vi "MICSD Status.vi"(0 "VISA Resource Name":refnum<visa-resource-name>, 11 "error in (no error)":errorcluster) -> (3 "Data Status":T1={"TX_BlockCount"=2650, "RX_BlockCount"=2650, "DataErrorCount"=2650}, 4 "dup VISA Resource Name":refnum<visa-resource-name>, 6 "Status Flags":T4, 8 "Link Status":T3={"ImplantID"=0, "CompanyID"=0, "RF_Channel"=4, "RX_Mod"=0, "TX_Mod"=0, "TXBlockSize"=15, "RXBlockSize"=15, "BlocksPerPack"=31} {"BlocksPerPack" items=["1"=1, "2"=2, "3"=3, "4"=4, "5"=5, "6"=6, "7"=7, "8"=8, "9"=9, "10"=10, "11"=11, "12"=12, "13"=13, "14"=14, "15"=15, "16"=16, "17"=17, "18"=18, "19"=19, "20"=20, "21"=21, "22"=22, "23"=23, "24"=24, "25"=25, "26"=26, "27"=27, "28"=28, "29"=29, "30"=30, "31"=31]; "RXBlockSize" items=["2"=2, "3"=3, "4"=4, "5"=5, "6"=6, "7"=7, "8"=8, "9"=9, "10"=10, "11"=11, "12"=12, "13"=13, "14"=14, "15"=15, "16"=16, "17"=17, "18"=18, "19"=19, "20"=20, "21"=21, "22"=22, "23"=23, "24"=24, "25"=25, "26"=26, "27"=27, "28"=28, "29"=29, "30"=30, "31"=31]; "TXBlockSize" items=["2"=2, "3"=3, "4"=4, "5"=5, "6"=6, "7"=7, "8"=8, "9"=9, "10"=10, "11"=11, "12"=12, "13"=13, "14"=14, "15"=15, "16"=16, "17"=17, "18"=18, "19"=19, "20"=20, "21"=21, "22"=22, "23"=23, "24"=24, "25"=25, "26"=26, "27"=27, "28"=28, "29"=29, "30"=30, "31"=31]; "TX_Mod" items=["2FSK-FB"=0, "2FSK"=2, "4FSK"=3]; "RX_Mod" items=["2FSK-FB"=0, "2FSK"=8, "4FSK"=12]; "RF_Channel" items=["0", "1", "2", "3", "4", "5", "6", "7", "8", "9"]; "CompanyID" format="%02x"; "ImplantID" format="%06x"}, 10 "Raw Status Data":u8[](array[numeric]), 14 "Link Quality":T2={"MAX_BIT_ERROR"=FALSE, "MAX_RETRIES"=FALSE, "Corrected Blocks"=2650, "CRC Errors"=2650}, 15 "error out":errorcluster)   [LabVIEW 2020]
uses:
  <vilib>/Instr/_visa.llb/VISA Configure Serial Port (Instr).vi
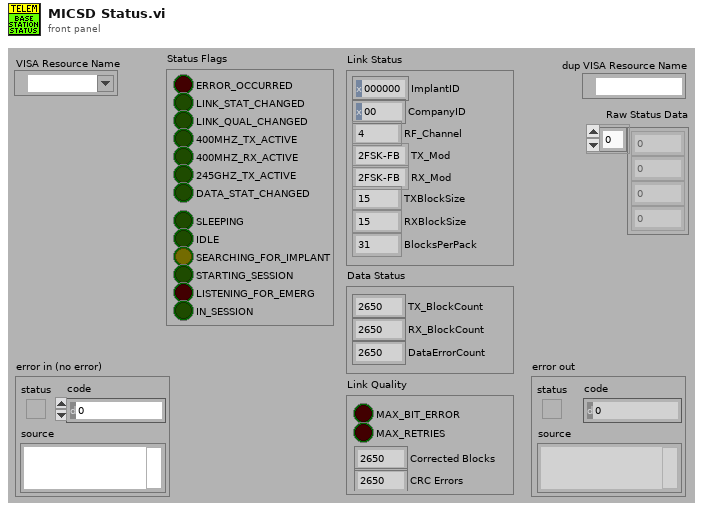
[diagram p1: front panel]
types:
  T1 = cluster{"TX_BlockCount":u16, "RX_BlockCount":u16, "DataErrorCount":u16}
  T2 = cluster{"MAX_BIT_ERROR":bool, "MAX_RETRIES":bool, "Corrected Blocks":u16, "CRC Errors":u16}
  T3 = cluster{"ImplantID":u32, "CompanyID":u8, "RF_Channel":u8, "RX_Mod":u8, "TX_Mod":u8, "TXBlockSize":u8, "RXBlockSize":u8, "BlocksPerPack":u8}
  T4 = cluster{"ERROR_OCCURRED":bool, "LINK_STAT_CHANGED":bool, "LINK_QUAL_CHANGED":bool, "400MHZ_TX_ACTIVE":bool, "400MHZ_RX_ACTIVE":bool, "245GHZ_TX_ACTIVE":bool, "DATA_STAT_CHANGED":bool, "SLEEPING":bool, "IDLE":bool, "SEARCHING_FOR_IMPLANT":bool, "STARTING_SESSION":bool, "LISTENING_FOR_EMERG":bool, "IN_SESSION":bool}
  T5 = cluster{"Command Token":u8, "Length":u16, "Pack Data":u8[]}
  T6 = cluster{"Read Data[0]":u8, "Read Data[1]":u8, "Read Data[2]":u8, "Read Data[3]":u8, "Read Data[4]":u8, "Read Data[5]":u8, "Read Data[6]":u8, "Read Data[7]":u8, "Read Data[8]":u8, "Read Data[9]":u8, "Read Data[10]":u8, "Read Data[11]":u8, "Read Data[12]":u8, "Read Data[13]":u8, "Read Data[14]":u8, "Read Data[15]":u8, "Read Data[16]":u8, "Read Data[17]":u8, "Read Data[18]":u8, "Read Data[19]":u8, "Read Data[20]":u8, "Read Data[21]":u8, "Read Data[22]":u8, "Read Data[23]":u8, "Read Data[24]":u8, "Read Data[25]":u8, "Read Data[26]":u8, "Read Data[27]":u8, "Read Data[28]":u8, "Read Data[29]":u8, "Read Data[30]":u8, "Read Data[31]":u8, "Read Data[32]":u8}
  T7 = cluster{"Boolean array[0]":bool, "Boolean array[1]":bool, "Boolean array[2]":bool, "Boolean array[3]":bool, "Boolean array[4]":bool, "Boolean array[5]":bool, "Boolean array[6]":bool, "Boolean array[7]":bool}
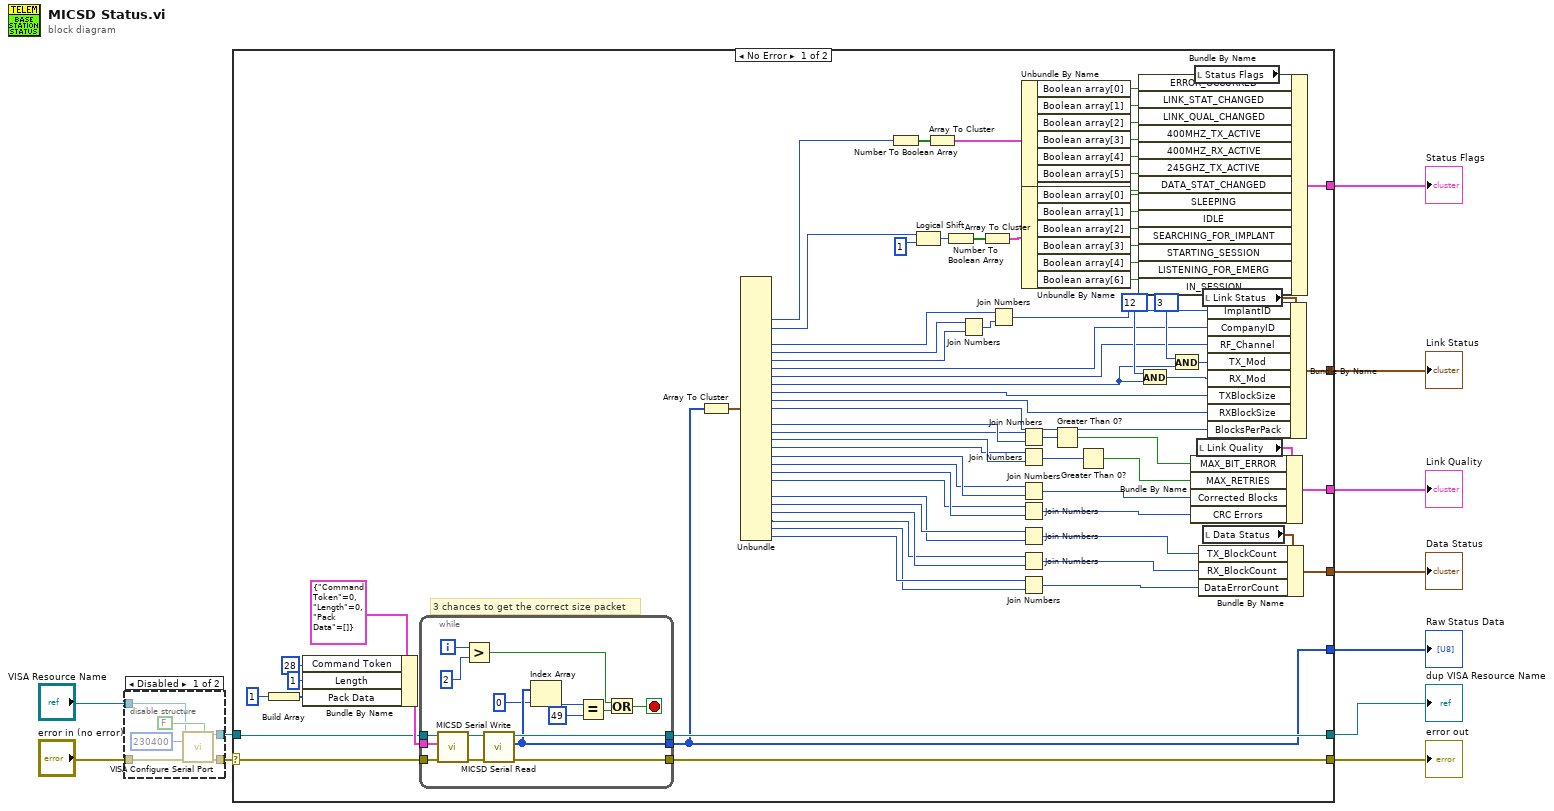
[diagram p0: block diagram]
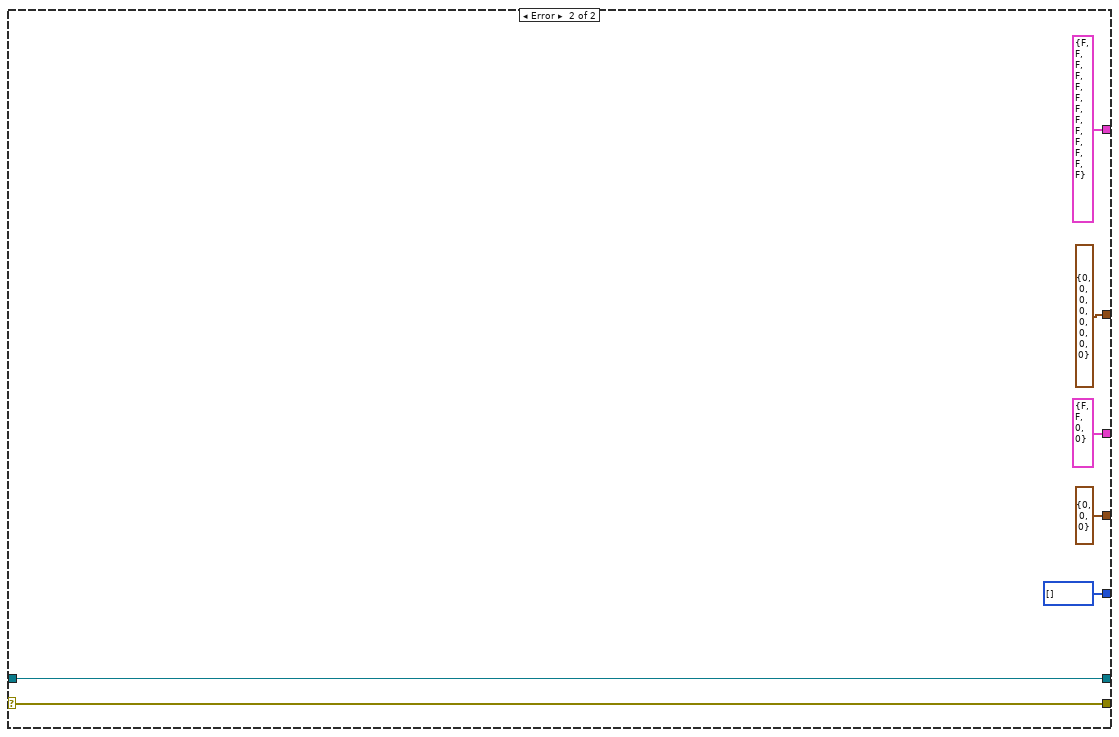
[diagram p3: hidden frame]
diagram:
  n1 = disable-structure shown="Disabled" {
    disable-tunnel: [w15 w18] -> w11
    disable-tunnel: [w14 w19] -> w10
    disable-tunnel: "VISA Resource Name" -> [w13 w19]
    disable-tunnel: "error in (no error)" -> [w12 w18]
    frame Disabled {
      n2 = call-poly "VISA Configure Serial Port"("VISA resource name"=w13, "Enable Termination\nChar (T)"=FALSE ("Enable Termination\nChar (T)"), "baud rate (9600)"=u32 230400, "error in (no error)"=w12) -> ("VISA resource name out"=w14:refnum<visa-resource-name>, "error out"=w15:errorcluster)  [unwired: 10 in]
    }
    frame Enabled {
    }
  }
  n3 = case shown="No Error" w11 {
    selector: w11 -> [w94 w121]
    tunnel: [w91 w121] -> w1
    tunnel: w10 -> [w93 w120]
    tunnel: [w92 w120] -> w7
    tunnel: [w89 T3 {"ImplantID"=0, "CompanyID"=0, "RF_Channel"=0, "RX_Mod"=0, "TX_Mod"=0, "TXBlockSize"=0, "RXBlockSize"=0, "BlocksPerPack"=0} ("Link Status")] -> w6
    tunnel: [w87 T4 {"ERROR_OCCURRED"=FALSE, "LINK_STAT_CHANGED"=FALSE, "LINK_QUAL_CHANGED"=FALSE, "400MHZ_TX_ACTIVE"=FALSE, "400MHZ_RX_ACTIVE"=FALSE, "245GHZ_TX_ACTIVE"=FALSE, "DATA_STAT_CHANGED"=FALSE, "SLEEPING"=FALSE, "IDLE"=FALSE, "SEARCHING_FOR_IMPLANT"=FALSE, "STARTING_SESSION"=FALSE, "LISTENING_FOR_EMERG"=FALSE, "IN_SESSION"=FALSE} ("Status Flags")] -> w5
    tunnel: [w85 T1 {"TX_BlockCount"=0, "RX_BlockCount"=0, "DataErrorCount"=0} ("Data Status")] -> w4
    tunnel: [w83 T2 {"MAX_BIT_ERROR"=FALSE, "MAX_RETRIES"=FALSE, "Corrected Blocks"=0, "CRC Errors"=0} ("Link Quality")] -> w3
    tunnel: [w61 u8[] [] ("Read Data")] -> w2
    frame No Error {
      # "3 chances to get the correct size packet"
      n4 = Build Array(u8 1 ("Length")) -> (w81:u8[])
      n5 = Bundle By Name(cluster=T5 {"Command Token"=0, "Length"=0, "Pack Data"=[]} ("Write Data"), "Command Token"=u8 28, "Length"=u16 1, "Pack Data"=w81) -> (w98:T5)
      n6 = while {
        tunnel: w98 -> [w114]
        tunnel: w94 -> [w112]
        tunnel: w93 -> [w111]
        tunnel: [w110] -> w92
        tunnel: [w109] -> w91
        tunnel: [w107] -> w61
        i -> [w101]
        stop <- w103 stop-if-true
        n7 = call "MICSD Serial Write.vi"("error in (no error)"=w112, "Write Data"=w114, "VISA Resource Name"=w111) -> ("error out"=w108:errorcluster, "DUP Visa Resource Name"=w113:refnum<visa-resource-name>)  [unwired: 7 in]
        n8 = Greater?(x=w101, y=2) -> (0:w99:bool)
        n9 = call "MICSD Serial Read.vi"("error in (no error)"=w108, "VISA Resource Name"=w113) -> ("error out"=w109:errorcluster, "Read Data"=w107:u8[], "DUP Visa Resource Name"=w110:refnum<visa-resource-name>)  [unwired: 7 in]
        n10 = Index Array(array=w107, index=0) -> (element=w105:u8)
        n11 = Equal?(x=w105, y=u8 49) -> (x = y?=w102:bool)
        n12 = Or(x=w99, y=w102) -> (x .or. y?=w103:bool)
      }
      n13 = Array To Cluster(array=w61) -> (cluster=w60:T6)
      n14 = Unbundle(w60) -> ("Read Data[5]"=w44:u8, "Read Data[6]"=w20:u8, "Read Data[8]"=w42:u8, "Read Data[9]"=w43:u8, "Read Data[10]"=w41:u8, "Read Data[11]"=w40:u8, "Read Data[12]"=w37:u8, "Read Data[13]"=w39:u8, "Read Data[14]"=w38:u8, "Read Data[15]"=w36:u8, "Read Data[16]"=w35:u8, "Read Data[18]"=w34:u8, "Read Data[19]"=w33:u8, "Read Data[20]"=w26:u8, "Read Data[21]"=w25:u8, "Read Data[22]"=w24:u8, "Read Data[23]"=w23:u8, "Read Data[24]"=w22:u8, "Read Data[25]"=w21:u8, "Read Data[27]"=w27:u8, "Read Data[28]"=w28:u8, "Read Data[29]"=w30:u8, "Read Data[30]"=w29:u8, "Read Data[31]"=w31:u8, "Read Data[32]"=w32:u8)  [unwired: 8 out]
      n15 = Number To Boolean Array(number=w44) -> (Boolean array=w80:bool[])
      n16 = Logical Shift(y=w20, x=u16 1 ("Length")) -> (x << y=w68:u16)
      n17 = Array To Cluster(array=w80) -> (cluster=w79:T7)
      n18 = Number To Boolean Array(number=w68) -> (Boolean array=w70:bool[])
      n19 = Join Numbers(hi=w43, lo=w41) -> ((hi.lo)=w59:u16)
      n20 = Array To Cluster(array=w70) -> (cluster=w69:T7)
      n21 = Join Numbers(hi=w42, lo=w59) -> ((hi.lo)=w58:u32)
      n22 = Join Numbers(hi=w33, lo=w34) -> ((hi.lo)=w52:u16)
      n23 = Join Numbers(hi=w25, lo=w26) -> ((hi.lo)=w53:u16)
      n24 = Join Numbers(hi=w23, lo=w24) -> ((hi.lo)=w49:u16)
      n25 = Join Numbers(hi=w21, lo=w22) -> ((hi.lo)=w48:u16)
      n26 = Join Numbers(hi=w28, lo=w27) -> ((hi.lo)=w47:u16)
      n27 = Join Numbers(hi=w29, lo=w30) -> ((hi.lo)=w46:u16)
      n28 = Join Numbers(hi=w32, lo=w31) -> ((hi.lo)=w45:u16)
      n29 = Unbundle By Name(w79) -> ("Boolean array[0]"=w78:bool, "Boolean array[1]"=w77:bool, "Boolean array[2]"=w76:bool, "Boolean array[3]"=w75:bool, "Boolean array[4]"=w74:bool, "Boolean array[5]"=w73:bool, "Boolean array[6]"=w72:bool)
      n30 = Unbundle By Name(w69) -> ("Boolean array[0]"=w67:bool, "Boolean array[1]"=w66:bool, "Boolean array[2]"=w65:bool, "Boolean array[3]"=w64:bool, "Boolean array[4]"=w63:bool, "Boolean array[6]"=w62:bool)
      n31 = Greater Than 0?(x=w52) -> (x > 0?=w51:bool)
      n32 = Greater Than 0?(x=w53) -> (x > 0?=w50:bool)
      n33 = And(x=u8 12 ("Command Token"), y=w39) -> (x .and. y?=w54:u8)
      n34 = And(x=u8 3 ("Command Token"), y=w39) -> (x .and. y?=w55:u8)
      n35 = local read "Status Flags"() -> (w88:T4)
      n36 = Bundle By Name(cluster=w88, "ERROR_OCCURRED"=w78, "LINK_STAT_CHANGED"=w77, "LINK_QUAL_CHANGED"=w76, "400MHZ_TX_ACTIVE"=w75, "400MHZ_RX_ACTIVE"=w74, "245GHZ_TX_ACTIVE"=w73, "DATA_STAT_CHANGED"=w72, "SLEEPING"=w67, "IDLE"=w66, "SEARCHING_FOR_IMPLANT"=w65, "STARTING_SESSION"=w64, "LISTENING_FOR_EMERG"=w63, "IN_SESSION"=w62) -> (w87:T4)
      n37 = local read "Link Quality"() -> (w84:T2)
      n38 = Bundle By Name(cluster=w84, "MAX_BIT_ERROR"=w51, "MAX_RETRIES"=w50, "Corrected Blocks"=w49, "CRC Errors"=w48) -> (w83:T2)
      n39 = local read "Link Status"() -> (w90:T3)
      n40 = local read "Data Status"() -> (w86:T1)
      n41 = Bundle By Name(cluster=w86, "TX_BlockCount"=w47, "RX_BlockCount"=w46, "DataErrorCount"=w45) -> (w85:T1)
      n42 = Bundle By Name(cluster=w90, "ImplantID"=w58, "CompanyID"=w40, "RF_Channel"=w37, "TX_Mod"=w55, "RX_Mod"=w54, "TXBlockSize"=w38, "RXBlockSize"=w36, "BlocksPerPack"=w35) -> (w89:T3)
    }
    frame Error {
    }
  }
  "dup VISA Resource Name" <- w7
  "error out" <- w1
  "Link Status" <- w6
  "Status Flags" <- w5
  "Data Status" <- w4
  "Link Quality" <- w3
  "Raw Status Data" <- w2
